vi "ReadAllFieldData.vi"(8 "error in (no error)":errorcluster, 11 "BME68x in":refnum<class "BME680.lvclass">) -> (0 "error out":errorcluster, 3 "BME68x out":refnum<class "BME680.lvclass">)   [LabVIEW 2022 SP3, in "BME680.lvlib" / "BME680.lvclass"]
uses:
  BME680.lvclass
  BME680.lvclass/BME680.ctl
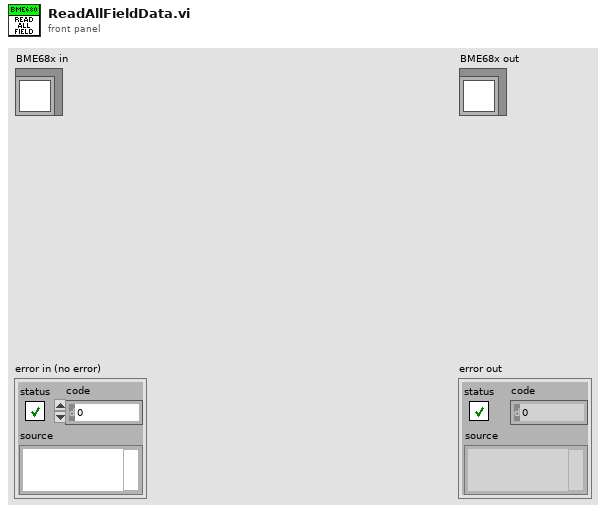
[diagram p1: front panel]
types:
  T1 = typedef "BME680.lvlib/BME680.lvclass/Data.ctl" = cluster{"Status":u8, "GasIdx":u8, "MeasIdx":u8, "ResHeat":u8, "iDac":u8, "GasWait":u8, "Temp":u16, "Pres":u32, "Hum":u8, "Gas Res":u8}
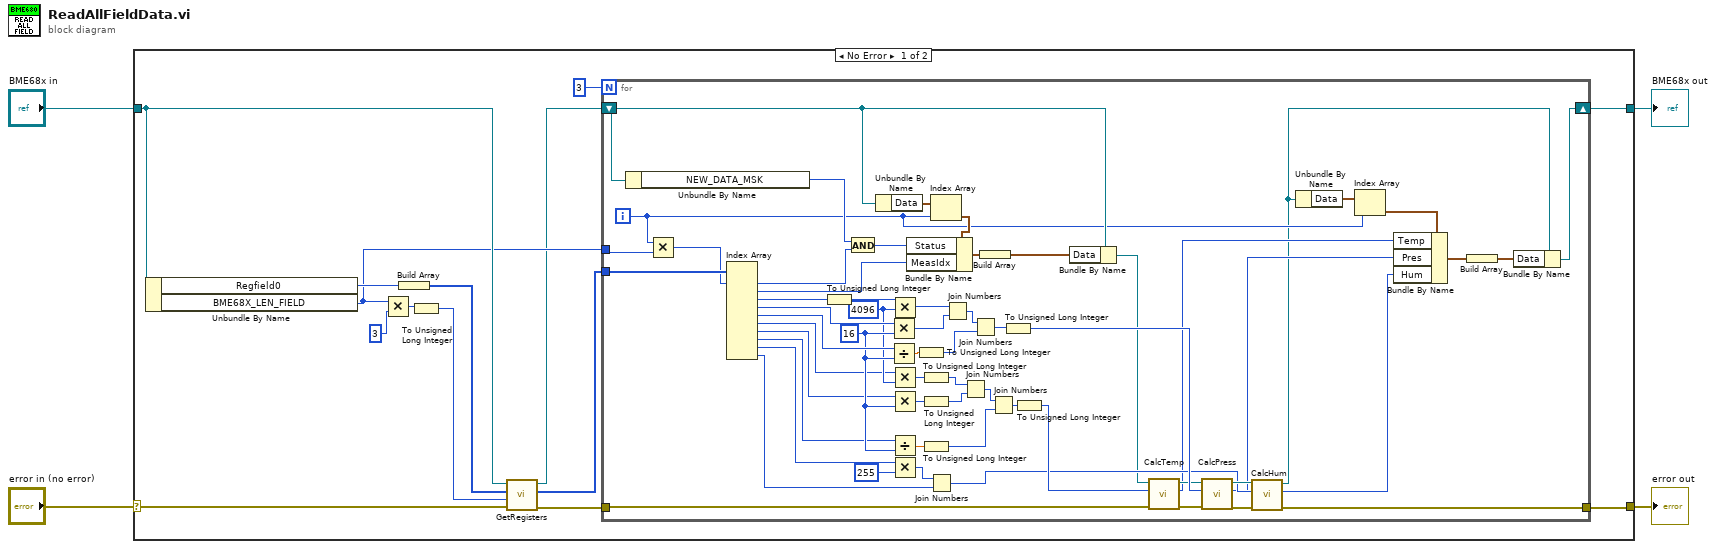
[diagram p0: block diagram]
diagram:
  n1 = case shown="No Error" "error in (no error)" {
    selector: "error in (no error)" -> [w18 w79]
    tunnel: [w7 w79] -> w3
    tunnel: [w5 w78] -> w1
    tunnel: "BME68x in" -> [w17 w78]
    frame No Error {
      n2 = Unbundle By Name(w17) -> ("Regfield0"=w16:u8, "BME68X_LEN_FIELD"=w9:u8)
      n3 = Multiply(x=w9, y=3) -> (x*y=w13:i32)
      n4 = Build Array(w16) -> (w15:u8[])
      n5 = To Unsigned Long Integer(number=w13) -> (unsigned 32bit integer=w12:u32)
      n6 = call-dynamic "GetRegisters.vi"("error in (no error)"=w18, "Lenght"=w12, "Addr"=w15, "BME680 in"=w17) -> ("error out"=w8:errorcluster, "Data out"=w11:u8[], "BME680 out"=w6:refnum<class "BME680.lvclass">)  [unwired: 5 in]
      n7 = for {
        N: 3 -> [_]
        tunnel: w11 -> [w76]
        tunnel: w9 -> [w77]
        tunnel: w8 -> [w40]
        tunnel: [w43] -> w7
        shift-right: [w19] -> w5
        shift-left: w6 -> [w32]
        i -> [w24]
        w61 = u8 16 ("y")
        w60 = u32 4096 ("y")
        n8 = Unbundle By Name(w32) -> ("NEW_DATA_MSK"=w73:u8)
        n9 = Multiply(x=w24, y=w77) -> (x*y=w75:i32)
        n10 = Index Array(array=w76, index #1=w75) -> (element #1=w72:u8, element #2=w74:u8, element #3=w70:u8, element #4=w69:u8, element #5=w67:u8, element #6=w59:u8, element #7=w58:u8, element #8=w57:u8, element #9=w53:u8, element #10=w44:u8)  [unwired: 9 in]
        n11 = To Unsigned Long Integer(number=w70) -> (unsigned 32bit integer=w68:u32)
        n12 = And(x=w73, y=w72) -> (x .and. y?=w71:u8)
        n13 = Unbundle By Name(w32) -> ("Data"=w34:T1[])
        n14 = Multiply(x=w69, y=w61) -> (x*y=w64:u8)
        n15 = Divide(x=w67, y=w61) -> (x/y=w66:dbl)
        n16 = Multiply(x=w68, y=w60) -> (x*y=w65:u32)
        n17 = Multiply(x=w59, y=w60) -> (x*y=w56:u32)
        n18 = Multiply(x=w58, y=w61) -> (x*y=w55:u8)
        n19 = Divide(x=w57, y=w61) -> (x/y=w54:dbl)
        n20 = Multiply(x=w53, y=u8 255) -> (x*y=w45:u8)
        n21 = To Unsigned Long Integer(number=w66) -> (unsigned 32bit integer=w63:u32)
        n22 = To Unsigned Long Integer(number=w56) -> (unsigned 32bit integer=w51:u32)
        n23 = To Unsigned Long Integer(number=w55) -> (unsigned 32bit integer=w50:u32)
        n24 = To Unsigned Long Integer(number=w54) -> (unsigned 32bit integer=w49:u32)
        n25 = Join Numbers(hi=w45, lo=w44) -> ((hi.lo)=w35:u16)
        n26 = Index Array(array=w34, index=w24) -> (element=w33:T1)
        n27 = Bundle By Name(cluster=w33, "Status"=w71, "MeasIdx"=w74) -> (w31:T1)
        n28 = Join Numbers(hi=w65, lo=w64) -> ((hi.lo)=w62:u64)
        n29 = Join Numbers(hi=w51, lo=w50) -> ((hi.lo)=w52:u64)
        n30 = Join Numbers(hi=w62, lo=w63) -> ((hi.lo)=w48:u64)
        n31 = Build Array(w31) -> (w30:T1[])
        n32 = Join Numbers(hi=w52, lo=w49) -> ((hi.lo)=w47:u64)
        n33 = To Unsigned Long Integer(number=w48) -> (unsigned 32bit integer=w39:u32)
        n34 = To Unsigned Long Integer(number=w47) -> (unsigned 32bit integer=w36:u32)
        n35 = Bundle By Name(cluster=w32, "Data"=w30) -> (w29:refnum<class "BME680.lvclass">)
        n36 = call "CalcTemp.vi"("error in (no error)"=w40, "Adc_temp"=w36, "BME68x in"=w29) -> ("error out"=w41:errorcluster, "Temp"=w21:i16, "BME68x out"=w38:refnum<class "BME680.lvclass">)  [unwired: 6 in]
        n37 = call "CalcPress.vi"("error in (no error)"=w41, "Adc_press"=w39, "BME68x in"=w38) -> ("error out"=w42:errorcluster, "Press"=w22:i32, "BME68x out"=w37:refnum<class "BME680.lvclass">)  [unwired: 6 in]
        n38 = call "CalcHum.vi"("error in (no error)"=w42, "Adc_Hum"=w35, "BME68x in"=w37) -> ("error out"=w43:errorcluster, "Hum"=w23:i32, "BME68x out"=w20:refnum<class "BME680.lvclass">)  [unwired: 6 in]
        n39 = Unbundle By Name(w20) -> ("Data"=w28:T1[])
        n40 = Index Array(array=w28, index=w24) -> (element=w27:T1)
        n41 = Bundle By Name(cluster=w27, "Temp"=w21, "Pres"=w22, "Hum"=w23) -> (w26:T1)
        n42 = Build Array(w26) -> (w25:T1[])
        n43 = Bundle By Name(cluster=w20, "Data"=w25) -> (w19:refnum<class "BME680.lvclass">)
      }
    }
    frame Error {
    }
  }
  "error out" <- w3
  "BME68x out" <- w1
